vi "migrate.vi"(8 "error in (no error)":errorcluster, 11 "plugin_interface in":refnum<class "lv-post-installer.lvclass">) -> (0 "error out":errorcluster, 3 "plugin_interface out":refnum<class "lv-post-installer.lvclass">)   [LabVIEW 2015, in "lv-post-installer.lvlib" / "lv-post-installer.lvclass"]
uses:
  lv-post-installer.lvclass
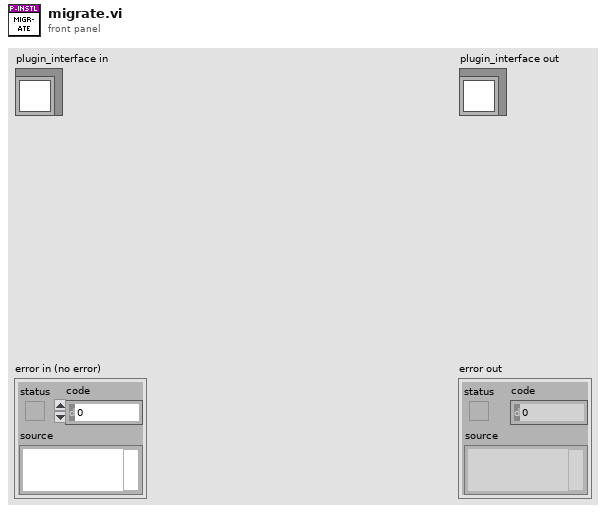
[diagram p1: front panel]
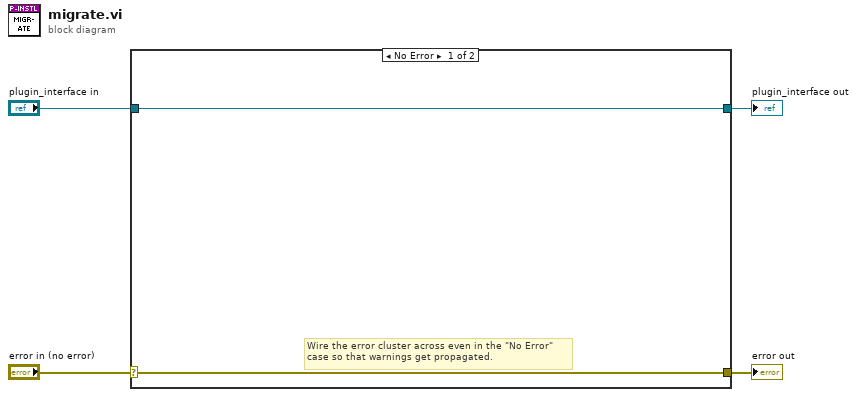
[diagram p0: block diagram]
diagram:
  n1 = case shown="No Error" "error in (no error)" {
    selector: "error in (no error)" -> [w5 w8]
    tunnel: [w5 w8] -> w3
    tunnel: [w6 w7] -> w1
    tunnel: "plugin_interface in" -> [w6 w7]
    frame No Error {
      # "Wire the error cluster across even in the \"No Error\"\ncase so that warnings get propagated."
    }
    frame Error {
    }
  }
  "error out" <- w3
  "plugin_interface out" <- w1
